vi "CRC check.vi"(1 "data IN":string) -> (0 "CRC fail":bool)   [LabVIEW 2010]
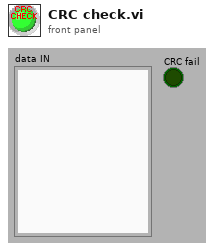
[diagram p1: front panel]
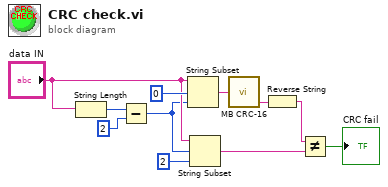
[diagram p0: block diagram]
diagram:
  n1 = String Length(string="data IN") -> (length=w3:i32)
  n2 = Subtract(x=w3, y=2) -> (x-y=w1:i32)
  n3 = String Subset(string="data IN", offset (0)=0, length (rest)=w1) -> (substring=w4:string)
  n4 = String Subset(string="data IN", offset (0)=w1, length (rest)=2 ("length (rest)")) -> (substring=w11:string)
  n5 = call "MB CRC-16.vi"("String"=w4) -> ("CRC-16"=w7:string)  [unwired: 2 in, 2 out]
  n6 = Reverse String(1:w7) -> (0:w10:string)
  n7 = Not Equal?(x=w10, y=w11) -> (x != y?=→"CRC fail":bool)
